vi "Flow High Limit SI.vi"(7 "Set? (F:Read)":bool, 8 "Error In":errorcluster, 9 "Flow High Limit (0 l/min)":dbl[unit], 10 "Channel (0)":i32, 11 "VISA resource name":refnum<visa-resource-name>) -> (0 "Error Out":errorcluster, 1 "Flow High Limit out":dbl[unit], 3 "dup VISA resource name":refnum<visa-resource-name>)   [LabVIEW 2016, in "MGC647C.lvlib"]
doc: "Read/Set flow high limit of a channel in SI unit."
uses:
  MGC647C.lvlib
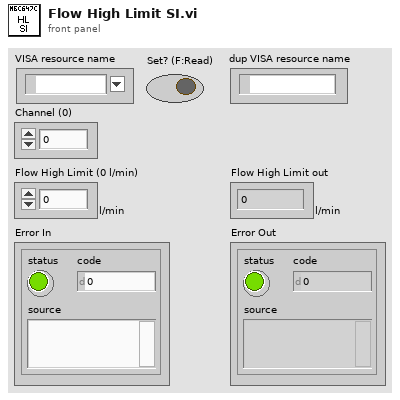
[diagram p1: front panel]
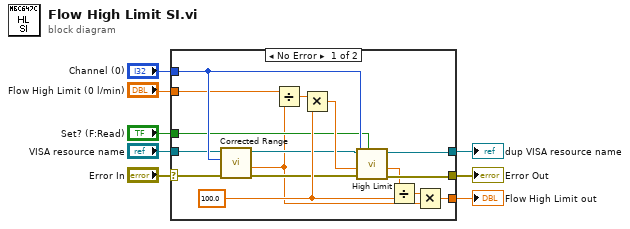
[diagram p0: block diagram]
diagram:
  n1 = case shown="No Error" "Error In" {
    selector: "Error In" -> [w16 w26]
    tunnel: "VISA resource name" -> [w11 w25]
    tunnel: [w24 w25] -> w7
    tunnel: [w23 w26] -> w6
    tunnel: "Set? (F:Read)" -> [w12 _]
    tunnel: "Flow High Limit (0 l/min)" -> [w10 w27]
    tunnel: [w20 w27] -> w2
    tunnel: "Channel (0)" -> [w13 _]
    frame No Error {
      w18 = 100.0 ("y")
      n2 = call "Corrected Range.vi"("Error In"=w16, "Channel (0)"=w13, "VISA resource name"=w11) -> ("Error Out"=w14:errorcluster, "Corrected Range"=w9:dbl[unit], "dup VISA resource name"=w15:refnum<visa-resource-name>)  [unwired: 6 in]
      n3 = Divide(x=w10, y=w9) -> (x/y=w19:dbl)
      n4 = Multiply(x=w19, y=w18) -> (x*y=w17:dbl)
      n5 = call "High Limit.vi"("Set? (F:Read)"=w12, "Error In"=w14, "High Limit (0%)"=w17, "Channel (0)"=w13, "VISA resource name"=w15) -> ("Error Out"=w23:errorcluster, "High Limit out"=w21:dbl, "dup VISA resource name"=w24:refnum<visa-resource-name>)  [unwired: 4 in]
      n6 = Divide(x=w21, y=w18) -> (x/y=w22:dbl)
      n7 = Multiply(x=w22, y=w9) -> (x*y=w20:dbl[unit])
    }
    frame Error {
    }
  }
  "dup VISA resource name" <- w7
  "Error Out" <- w6
  "Flow High Limit out" <- w2
